vi "Read Single Measurement.vi"(8 "error in (no error)":errorcluster, 11 "VISA resource name":refnum<visa-resource-name>) -> (0 "error out":errorcluster, 2 "Measurement":dbl format="%#.10g", 3 "VISA resource name out":refnum<visa-resource-name>)   [LabVIEW 2012, in "Fluke 8508.lvlib"]
doc: "This VI reads and returns a single measurement from the instrument. The measurement read is the last triggered reading. \n\nNOTE: If the triggering mode is set to \"external\" and a delay is set in \"Configure Trigger\", it may be possible to get an incorrect reading if the delay time has not elapsed before taking a reading since the measurement returned will the be the one from the previous trigger.\n\nNOTE: In some measurement modes, the instruments will timeout before the measurement is complete. For instance, a single measurement can take up to two minutes while the devide is in true ohms mode and configured for an 8 1/2 digit reading. If you run into this problem, set the timeout as necessary using the set timeout VI in the VISA palette."
uses:
  Fluke 8508.lvlib
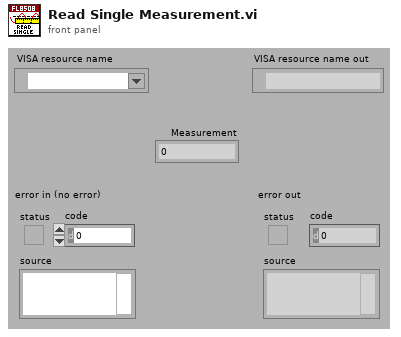
[diagram p1: front panel]
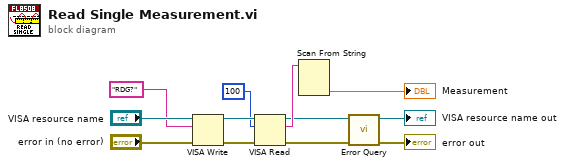
[diagram p0: block diagram]
diagram:
  n1 = VISA Write(VISA resource name="VISA resource name", write buffer="RDG?", error in (no error)="error in (no error)") -> (VISA resource name out=w11:refnum<visa-resource-name>, error out=w12:errorcluster)  [unwired: 1 out]
  n2 = VISA Read(VISA resource name=w11, byte count=u32 100, error in (no error)=w12) -> (VISA resource name out=w2:refnum<visa-resource-name>, read buffer=w6:string, error out=w4:errorcluster)  [unwired: 1 out]
  n3 = Scan From String(input string=w6) -> (output 1=→"Measurement":dbl)  [unwired: 4 in, 3 out]
  n4 = call "Error Query.vi"("error in (no error)"=w4, "VISA resource name"=w2) -> ("error out"=→"error out":errorcluster, "VISA resource name out"=→"VISA resource name out":refnum<visa-resource-name>)  [unwired: 6 in, 2 out]
